vi "get active image from buffer.vi"(8 "error in (no error)":errorcluster, 11 "Thorcam in":refnum<class "Thorcam.lvclass">) -> (0 "error out":errorcluster, 2 "Image Memory Out":u8[](array[numeric]), 3 "Thorcam out":refnum<class "Thorcam.lvclass">)   [LabVIEW 2012, in "Thorcam.lvclass"]
uses:
  Thorcam.lvclass
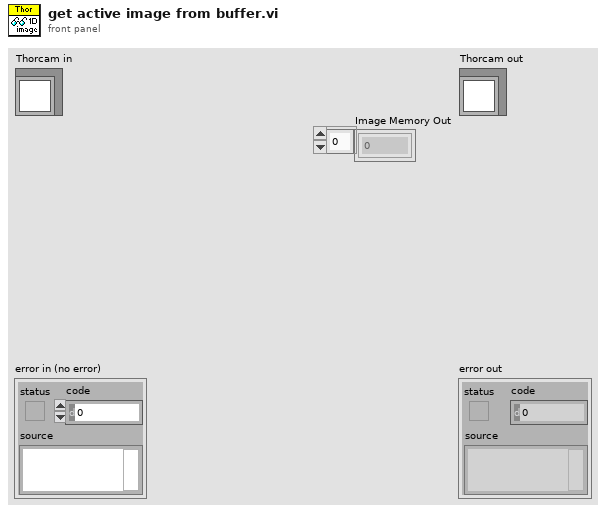
[diagram p1: front panel]
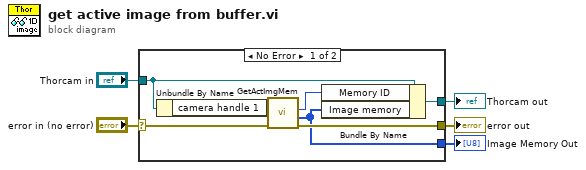
[diagram p0: block diagram]
diagram:
  n1 = case shown="No Error" "error in (no error)" {
    selector: "error in (no error)" -> [w11 w14]
    tunnel: [w10 w14] -> w4
    tunnel: [w7 w13] -> w2
    tunnel: "Thorcam in" -> [w8 w13]
    tunnel: [w6 _] -> w1
    frame No Error {
      n2 = Unbundle By Name(w8) -> ("camera handle 1"=w12:u32)
      n3 = call <instrlib>:"GetActImgMem.vi"("error in"=w11, "Camera Handle In"=w12) -> ("error out"=w10:errorcluster, "Image Memory Out"=w6:u8[], "Memory Number"=w9:i32)  [unwired: 6 in, 1 out]
      n4 = Bundle By Name(cluster=w8, "Memory ID"=w9, "Image memory"=w6) -> (w7:refnum<class "Thorcam.lvclass">)
    }
    frame Error {
    }
  }
  "error out" <- w4
  "Thorcam out" <- w2
  "Image Memory Out" <- w1
